vi "Do.vi"(8 "error in (no error)":errorcluster, 10 "Actor in":refnum<class "Actor.lvclass">, 11 "Recieve New Subscription Msg":refnum<class "Recieve New Subscription Msg.lvclass">) -> (0 "error out":errorcluster, 2 "Actor out":refnum<class "Actor.lvclass">)   [LabVIEW 2020, in "Actor Pub Sub Channels.lvlib" / "Recieve New Subscription Msg.lvclass"]
doc: "This VI delivers the message to the actor by calling the appropriate method(s) on the actor."
uses:
  Recieve New Subscription Msg.lvclass
  <vilib>/ActorFramework/Actor/Actor.lvclass
  Recieve New Subscription Msg.lvclass/Recieve New Subscription Msg.ctl
  PubSub Status Reciever Interface/PubSub Status Reciever Interface.lvclass
  9ef47adc-f318-494c-9b8b-6df3216d6863.vi
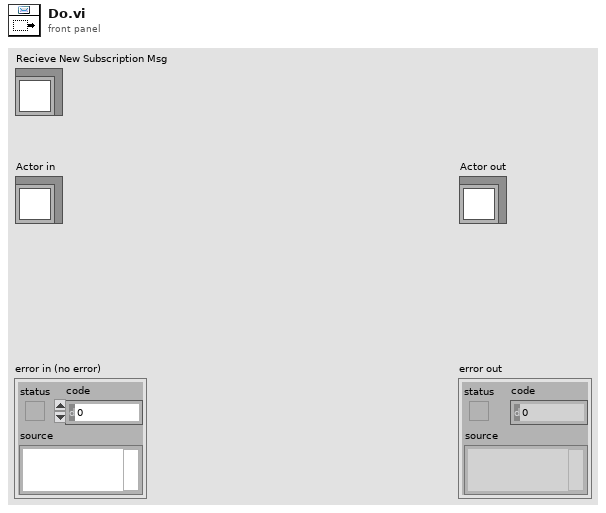
[diagram p1: front panel]
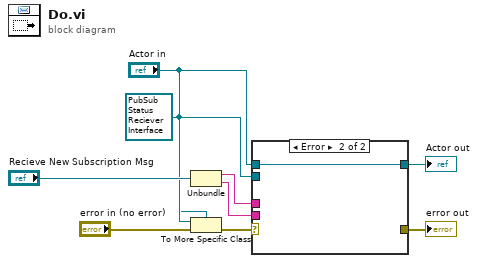
[diagram p0: block diagram]
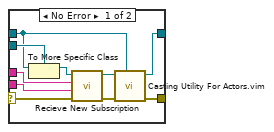
[diagram p2: hidden frame]
diagram:
  w3 = refnum<class "PubSub Status Reciever Interface.lvclass"> refnum ("Actor in")
  n1 = Unbundle("Recieve New Subscription Msg") -> (w2:string, w1:string)
  n2 = To More Specific Class(target class=w3, reference="Actor in", error in="error in (no error)") -> (error out=w7:errorcluster)  [unwired: 1 out]
  n3 = case shown="Error" w7 {
    selector: w7 -> [w19 _]
    tunnel: [w13 _] -> w6
    tunnel: [w14 w20] -> w5
    tunnel: "Actor in" -> [w16 w20]
    tunnel: w3 -> [w17 _]
    tunnel: w2 -> [w11 _]
    tunnel: w1 -> [w10 _]
    frame No Error {
      n4 = To More Specific Class(target class=w17, reference=w16) -> (specific class reference=w18:refnum<class "PubSub Status Reciever Interface.lvclass">)  [unwired: 1 in, 1 out]
      n5 = call-dynamic "Recieve New Subscription.vi"("error in (no error)"=w19, "Topic"=w10, "Name"=w11, "PubSub Status Reciever Interface in"=w18) -> ("error out"=w12:errorcluster, "PubSub Status Reciever Interface out"=w15:refnum<class "PubSub Status Reciever Interface.lvclass">)  [unwired: 6 in]
      n6 = call "Casting Utility For Actors.vim"("type"=w16, "error in (no error)"=w12, "Actor in"=w15) -> ("error out"=w13:errorcluster, "Actor out"=w14:refnum<class "Actor.lvclass">)  [unwired: 7 in]
    }
    frame Error {
    }
  }
  "error out" <- w6
  "Actor out" <- w5
